vi "Read read operation timeout.vi"(8 "error in (no error)":errorcluster, 11 "transmission data unit in":refnum<class "Transmission Data Unit.lvclass">) -> (0 "error out":errorcluster, 2 "read operation timeout":i32, 3 "transmission data unit out":refnum<class "Transmission Data Unit.lvclass">)   [LabVIEW 2020, in "SubVIs.lvlib" / "Transmission Data Unit.lvclass"]
uses:
  <vilib>/Modbus/subvis/Transmission Data Unit (ADU)/Transmission Data Unit/Transmission Data Unit.lvclass
  <vilib>/Modbus/subvis/Transmission Data Unit (ADU)/Transmission Data Unit/Transmission Data Unit.lvclass/Transmission Data Unit.ctl
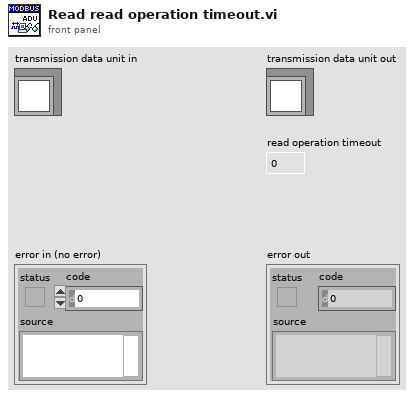
[diagram p1: front panel]
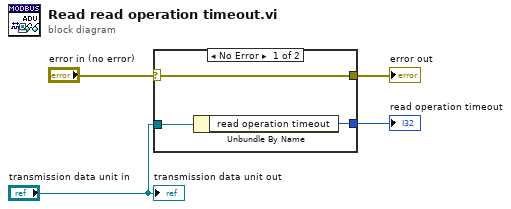
[diagram p0: block diagram]
diagram:
  n1 = case shown="No Error" "error in (no error)" {
    selector: "error in (no error)" -> [w5 w8]
    tunnel: "transmission data unit in" -> [w7 _]
    tunnel: [w6 _] -> w3
    tunnel: [w5 w8] -> w1
    frame No Error {
      n2 = Unbundle By Name(w7) -> ("read operation timeout"=w6:i32)
    }
    frame Error {
    }
  }
  "error out" <- w1
  "read operation timeout" <- w3
  "transmission data unit out" <- "transmission data unit in"
